vi "Plot Update Cursor 2D Table.vi"(6 "Cursor XYZ":T1, 8 "Data 2D Table":cluster{"X":sgl[], "Y":sgl[], "Z":sgl[][]}, 11 "Table Ref":refnum<vi>) -> ()   [LabVIEW 2016]
uses:
  <vilib>/addons/Software Calibration Management/xSCM/Controls/TLU2D.ctl
  <vilib>/Utility/miscctls.llb/LVRowAndColumnTypeDef.ctl
  <vilib>/addons/Software Calibration Management/xSCM/SCM-API.lvlib
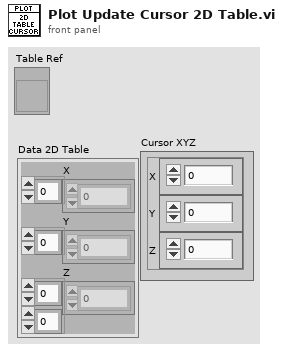
[diagram p1: front panel]
types:
  T1 = typedef "SCM-API.lvlib/TLU2D.ctl" = cluster{"X":sgl, "Y":sgl, "Z":sgl}
  T2 = typedef "LVRowAndColumnTypeDef.ctl" = cluster{"Row":i32, "Column":i32}
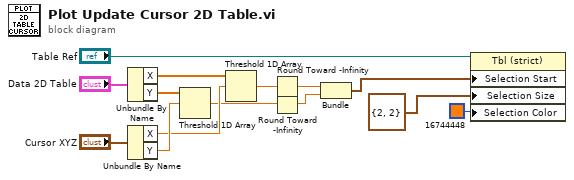
[diagram p0: block diagram]
diagram:
  n1 = Unbundle By Name("Data 2D Table") -> ("X"=w10:sgl[], "Y"=w12:sgl[])
  n2 = Unbundle By Name("Cursor XYZ") -> ("X"=w9:sgl, "Y"=w11:sgl)
  n3 = Threshold 1D Array(2:w11, 3:w12) -> (0:w7:sgl)  [unwired: 1 in]
  n4 = Threshold 1D Array(2:w9, 3:w10) -> (0:w8:sgl)  [unwired: 1 in]
  n5 = Round Toward -Infinity(1:w8) -> (0:w4:sgl)
  n6 = Round Toward -Infinity(1:w7) -> (0:w3:sgl)
  n7 = Bundle(w4, w3) -> (w2:cluster{sgl, sgl})  [unwired: 1 in]
  n8 = property on="Property Node" class="Tbl (strict)"(reference="Table Ref", "Selection Start"=w2, "Selection Size"=T2 {"Row"=2, "Column"=2}, "Selection Color"=u32 16744448) -> ()  [unwired: 1 in, 2 out]
